vi "IdentifyChange.vi"(8 "error in (no error)":errorcluster, 9 "NewVal":T2 {"Hardware"."Logical Instrument"."Watchdog"."Interval (s)" min=1.0 max=360.0; "Hardware"."Logical Instrument"."Safety Trips"."Pmax Sink Time (s)" min=-1.0; "Hardware"."Logical Instrument"."Safety Trips"."Pmax Sink (W)" min=0.0 format="%#_7g"; "Hardware"."Logical Instrument"."Safety Trips"."Pmax Source Time (s)" min=-1.0; "Hardware"."Logical Instrument"."Safety Trips"."Pmax Source (W)" min=0.0 format="%#_7g"; "Hardware"."Logical Instrument"."Safety Trips"."Absolute Curr Peak" min=0.0; "Hardware"."Logical Instrument"."Safety Trips"."Imax Sink Time (s)" min=-1.0; "Hardware"."Logical Instrument"."Safety Trips"."Imax Sink (A)" min=0.0; "Hardware"."Logical Instrument"."Safety Trips"."Imax Source Time (s)" min=-1.0; "Hardware"."Logical Instrument"."Safety Trips"."Imax Source (A)" min=0.0; "Hardware"."Logical Instrument"."Safety Trips"."Absolute Volt Peak" min=0.0; "Hardware"."Logical Instrument"."Safety Trips"."Vmax Time (s)" min=-1.0; "Hardware"."Logical Instrument"."Safety Trips"."Vmax (V)" min=0.0; "Hardware"."Logical Instrument"."Safety Trips"."Vmin Time (s)" min=-1.0; "Hardware"."Logical Instrument"."Safety Trips"."Vmin (V)" min=0.0; "Hardware"."Logical Instrument"."Aperture (cycles)" min=1 max=64; "Hardware"."Logical Instrument"."FreqOut (Hz)" min=0.0 max=100.0; "Hardware"."Logical Instrument"."Slew Rates"."Phase Angle Min (Deg/s)" min=0.0; "Hardware"."Logical Instrument"."Slew Rates"."Phase Angle Max (Deg/s)" min=0.0; "Hardware"."Logical Instrument"."Slew Rates"."Freq Min (Hz/s)" min=0.0; "Hardware"."Logical Instrument"."Slew Rates"."Freq Max (Hz/s)" min=0.0; "Hardware"."Logical Instrument"."Slew Rates"."Pmax (W/s)" min=0.0; "Hardware"."Logical Instrument"."Slew Rates"."Pmin (W/s)" min=0.0; "Hardware"."Logical Instrument"."Slew Rates"."Imax (A/s)" min=0.0; "Hardware"."Logical Instrument"."Slew Rates"."Vmax (V/s)" min=0.0; "Hardware"."Logical Instrument"."Slew Rates"."Imin (A/s)" min=0.0; "Hardware"."Logical Instrument"."Slew Rates"."Vmin (V/s)" min=0.0; "Hardware"."Logical Instrument"."Phases"."Change at (Deg)" min=0.0; "Hardware"."Logical Instrument"."Phases"."C-Angle (Deg)" min=0.0; "Hardware"."Logical Instrument"."Phases"."B-Angle (Deg)" min=0.0; "Hardware"."Logical Instrument"."Phases"."C-Volts (V)" min=0.0; "Hardware"."Logical Instrument"."Phases"."B-Volts (V)" min=0.0; "Hardware"."Logical Instrument"."Phases"."A-Volts (V)" min=0.0; "Hardware"."Logical Instrument"."Vout (V)" min=0.0; "Hardware"."Mode" items=["3-Phase AC"=0, "AC"=1, "DC"=2, "AC - AC"=7, "AC - DC"=8, "DC - AC"=11, "DC - DC"=12, "2-Phase AC - AC"=5, "2-Phase AC - DC"=6, "AC - AC - AC"=3, "DC - DC - DC"=4, "AC - AC - DC"=9, "AC - DC - DC"=10, "AC - DC - AC"=13, "DC - AC - AC"=14, "DC - AC - DC"=15]}, 10 "OldVal":T2 {"Hardware"."Logical Instrument"."Watchdog"."Interval (s)" min=1.0 max=360.0; "Hardware"."Logical Instrument"."Safety Trips"."Pmax Sink Time (s)" min=-1.0; "Hardware"."Logical Instrument"."Safety Trips"."Pmax Sink (W)" min=0.0 format="%#_7g"; "Hardware"."Logical Instrument"."Safety Trips"."Pmax Source Time (s)" min=-1.0; "Hardware"."Logical Instrument"."Safety Trips"."Pmax Source (W)" min=0.0 format="%#_7g"; "Hardware"."Logical Instrument"."Safety Trips"."Absolute Curr Peak" min=0.0; "Hardware"."Logical Instrument"."Safety Trips"."Imax Sink Time (s)" min=-1.0; "Hardware"."Logical Instrument"."Safety Trips"."Imax Sink (A)" min=0.0; "Hardware"."Logical Instrument"."Safety Trips"."Imax Source Time (s)" min=-1.0; "Hardware"."Logical Instrument"."Safety Trips"."Imax Source (A)" min=0.0; "Hardware"."Logical Instrument"."Safety Trips"."Absolute Volt Peak" min=0.0; "Hardware"."Logical Instrument"."Safety Trips"."Vmax Time (s)" min=-1.0; "Hardware"."Logical Instrument"."Safety Trips"."Vmax (V)" min=0.0; "Hardware"."Logical Instrument"."Safety Trips"."Vmin Time (s)" min=-1.0; "Hardware"."Logical Instrument"."Safety Trips"."Vmin (V)" min=0.0; "Hardware"."Logical Instrument"."Aperture (cycles)" min=1 max=64; "Hardware"."Logical Instrument"."FreqOut (Hz)" min=0.0 max=100.0; "Hardware"."Logical Instrument"."Slew Rates"."Phase Angle Min (Deg/s)" min=0.0; "Hardware"."Logical Instrument"."Slew Rates"."Phase Angle Max (Deg/s)" min=0.0; "Hardware"."Logical Instrument"."Slew Rates"."Freq Min (Hz/s)" min=0.0; "Hardware"."Logical Instrument"."Slew Rates"."Freq Max (Hz/s)" min=0.0; "Hardware"."Logical Instrument"."Slew Rates"."Pmax (W/s)" min=0.0; "Hardware"."Logical Instrument"."Slew Rates"."Pmin (W/s)" min=0.0; "Hardware"."Logical Instrument"."Slew Rates"."Imax (A/s)" min=0.0; "Hardware"."Logical Instrument"."Slew Rates"."Vmax (V/s)" min=0.0; "Hardware"."Logical Instrument"."Slew Rates"."Imin (A/s)" min=0.0; "Hardware"."Logical Instrument"."Slew Rates"."Vmin (V/s)" min=0.0; "Hardware"."Logical Instrument"."Phases"."Change at (Deg)" min=0.0; "Hardware"."Logical Instrument"."Phases"."C-Angle (Deg)" min=0.0; "Hardware"."Logical Instrument"."Phases"."B-Angle (Deg)" min=0.0; "Hardware"."Logical Instrument"."Phases"."C-Volts (V)" min=0.0; "Hardware"."Logical Instrument"."Phases"."B-Volts (V)" min=0.0; "Hardware"."Logical Instrument"."Phases"."A-Volts (V)" min=0.0; "Hardware"."Logical Instrument"."Vout (V)" min=0.0; "Hardware"."Mode" items=["3-Phase AC"=0, "AC"=1, "DC"=2, "AC - AC"=7, "AC - DC"=8, "DC - AC"=11, "DC - DC"=12, "2-Phase AC - AC"=5, "2-Phase AC - DC"=6, "AC - AC - AC"=3, "DC - DC - DC"=4, "AC - AC - DC"=9, "AC - DC - DC"=10, "AC - DC - AC"=13, "DC - AC - AC"=14, "DC - AC - DC"=15]}, 11 "Settings In":T2 {"Hardware"."Logical Instrument"."Watchdog"."Interval (s)" min=1.0 max=360.0; "Hardware"."Logical Instrument"."Safety Trips"."Pmax Sink Time (s)" min=-1.0; "Hardware"."Logical Instrument"."Safety Trips"."Pmax Sink (W)" min=0.0 format="%#_7g"; "Hardware"."Logical Instrument"."Safety Trips"."Pmax Source Time (s)" min=-1.0; "Hardware"."Logical Instrument"."Safety Trips"."Pmax Source (W)" min=0.0 format="%#_7g"; "Hardware"."Logical Instrument"."Safety Trips"."Absolute Curr Peak" min=0.0; "Hardware"."Logical Instrument"."Safety Trips"."Imax Sink Time (s)" min=-1.0; "Hardware"."Logical Instrument"."Safety Trips"."Imax Sink (A)" min=0.0; "Hardware"."Logical Instrument"."Safety Trips"."Imax Source Time (s)" min=-1.0; "Hardware"."Logical Instrument"."Safety Trips"."Imax Source (A)" min=0.0; "Hardware"."Logical Instrument"."Safety Trips"."Absolute Volt Peak" min=0.0; "Hardware"."Logical Instrument"."Safety Trips"."Vmax Time (s)" min=-1.0; "Hardware"."Logical Instrument"."Safety Trips"."Vmax (V)" min=0.0; "Hardware"."Logical Instrument"."Safety Trips"."Vmin Time (s)" min=-1.0; "Hardware"."Logical Instrument"."Safety Trips"."Vmin (V)" min=0.0; "Hardware"."Logical Instrument"."Aperture (cycles)" min=1 max=64; "Hardware"."Logical Instrument"."FreqOut (Hz)" min=0.0 max=100.0; "Hardware"."Logical Instrument"."Slew Rates"."Phase Angle Min (Deg/s)" min=0.0; "Hardware"."Logical Instrument"."Slew Rates"."Phase Angle Max (Deg/s)" min=0.0; "Hardware"."Logical Instrument"."Slew Rates"."Freq Min (Hz/s)" min=0.0; "Hardware"."Logical Instrument"."Slew Rates"."Freq Max (Hz/s)" min=0.0; "Hardware"."Logical Instrument"."Slew Rates"."Pmax (W/s)" min=0.0; "Hardware"."Logical Instrument"."Slew Rates"."Pmin (W/s)" min=0.0; "Hardware"."Logical Instrument"."Slew Rates"."Imax (A/s)" min=0.0; "Hardware"."Logical Instrument"."Slew Rates"."Vmax (V/s)" min=0.0; "Hardware"."Logical Instrument"."Slew Rates"."Imin (A/s)" min=0.0; "Hardware"."Logical Instrument"."Slew Rates"."Vmin (V/s)" min=0.0; "Hardware"."Logical Instrument"."Phases"."Change at (Deg)" min=0.0; "Hardware"."Logical Instrument"."Phases"."C-Angle (Deg)" min=0.0; "Hardware"."Logical Instrument"."Phases"."B-Angle (Deg)" min=0.0; "Hardware"."Logical Instrument"."Phases"."C-Volts (V)" min=0.0; "Hardware"."Logical Instrument"."Phases"."B-Volts (V)" min=0.0; "Hardware"."Logical Instrument"."Phases"."A-Volts (V)" min=0.0; "Hardware"."Logical Instrument"."Vout (V)" min=0.0; "Hardware"."Mode" items=["3-Phase AC"=0, "AC"=1, "DC"=2, "AC - AC"=7, "AC - DC"=8, "DC - AC"=11, "DC - DC"=12, "2-Phase AC - AC"=5, "2-Phase AC - DC"=6, "AC - AC - AC"=3, "DC - DC - DC"=4, "AC - AC - DC"=9, "AC - DC - DC"=10, "AC - DC - AC"=13, "DC - AC - AC"=14, "DC - AC - DC"=15]}) -> (0 "error out":errorcluster, 1 "Instrument Index":i32, 2 "Ctrl Label":string, 3 "Settings Out":T2 {"Hardware"."Logical Instrument"."Watchdog"."Interval (s)" min=1.0 max=360.0; "Hardware"."Logical Instrument"."Safety Trips"."Pmax Sink Time (s)" min=-1.0; "Hardware"."Logical Instrument"."Safety Trips"."Pmax Sink (W)" min=0.0 format="%#_7g"; "Hardware"."Logical Instrument"."Safety Trips"."Pmax Source Time (s)" min=-1.0; "Hardware"."Logical Instrument"."Safety Trips"."Pmax Source (W)" min=0.0 format="%#_7g"; "Hardware"."Logical Instrument"."Safety Trips"."Absolute Curr Peak" min=0.0; "Hardware"."Logical Instrument"."Safety Trips"."Imax Sink Time (s)" min=-1.0; "Hardware"."Logical Instrument"."Safety Trips"."Imax Sink (A)" min=0.0; "Hardware"."Logical Instrument"."Safety Trips"."Imax Source Time (s)" min=-1.0; "Hardware"."Logical Instrument"."Safety Trips"."Imax Source (A)" min=0.0; "Hardware"."Logical Instrument"."Safety Trips"."Absolute Volt Peak" min=0.0; "Hardware"."Logical Instrument"."Safety Trips"."Vmax Time (s)" min=-1.0; "Hardware"."Logical Instrument"."Safety Trips"."Vmax (V)" min=0.0; "Hardware"."Logical Instrument"."Safety Trips"."Vmin Time (s)" min=-1.0; "Hardware"."Logical Instrument"."Safety Trips"."Vmin (V)" min=0.0; "Hardware"."Logical Instrument"."Aperture (cycles)" min=1 max=64; "Hardware"."Logical Instrument"."FreqOut (Hz)" min=0.0 max=100.0; "Hardware"."Logical Instrument"."Slew Rates"."Phase Angle Min (Deg/s)" min=0.0; "Hardware"."Logical Instrument"."Slew Rates"."Phase Angle Max (Deg/s)" min=0.0; "Hardware"."Logical Instrument"."Slew Rates"."Freq Min (Hz/s)" min=0.0; "Hardware"."Logical Instrument"."Slew Rates"."Freq Max (Hz/s)" min=0.0; "Hardware"."Logical Instrument"."Slew Rates"."Pmax (W/s)" min=0.0; "Hardware"."Logical Instrument"."Slew Rates"."Pmin (W/s)" min=0.0; "Hardware"."Logical Instrument"."Slew Rates"."Imax (A/s)" min=0.0; "Hardware"."Logical Instrument"."Slew Rates"."Vmax (V/s)" min=0.0; "Hardware"."Logical Instrument"."Slew Rates"."Imin (A/s)" min=0.0; "Hardware"."Logical Instrument"."Slew Rates"."Vmin (V/s)" min=0.0; "Hardware"."Logical Instrument"."Phases"."Change at (Deg)" min=0.0; "Hardware"."Logical Instrument"."Phases"."C-Angle (Deg)" min=0.0; "Hardware"."Logical Instrument"."Phases"."B-Angle (Deg)" min=0.0; "Hardware"."Logical Instrument"."Phases"."C-Volts (V)" min=0.0; "Hardware"."Logical Instrument"."Phases"."B-Volts (V)" min=0.0; "Hardware"."Logical Instrument"."Phases"."A-Volts (V)" min=0.0; "Hardware"."Logical Instrument"."Vout (V)" min=0.0; "Hardware"."Mode" items=["3-Phase AC"=0, "AC"=1, "DC"=2, "AC - AC"=7, "AC - DC"=8, "DC - AC"=11, "DC - DC"=12, "2-Phase AC - AC"=5, "2-Phase AC - DC"=6, "AC - AC - AC"=3, "DC - DC - DC"=4, "AC - AC - DC"=9, "AC - DC - DC"=10, "AC - DC - AC"=13, "DC - AC - AC"=14, "DC - AC - DC"=15]})   [LabVIEW 2018, in "AcPwrPlugins.lvlib" / "NHRGridSim.lvclass"]
doc: "When the user makes any changes in the NHRGrid \"Settings\", this VI identifies which specific control was changed, and from which logical instrument."
uses:
  NHRGridSim.lvclass
  TypeDefs/NHRGrid_Device(s)Settings.ctl
  TypeDefs/NHRGrid_Hardware.ctl
  TypeDefs/NHRGrid_Modes.ctl
  TypeDefs/NHRGrid_Logical_Instrument.ctl
  TypeDefs/NHRGrid_InstrumentCluster.ctl
  TypeDefs/NHRGrid_Phases.ctl
  TypeDefs/NHRGrid_SlewRates.ctl
  TypeDefs/NHRGrid_Ranges.ctl
  TypeDefs/NHRGrid_SafetyTrips.ctl
  TypeDefs/NHRGrid_Watchdog.ctl
  TypeDefs/NHRGrid_ItemCheck.ctl
panel:
  in  "Tab Control":T1(tab)
  # "Voltages (L-N)"
  # "Voltages (L-N)"
  # "Voltages (L-N)"
  # "Voltages (L-N)"
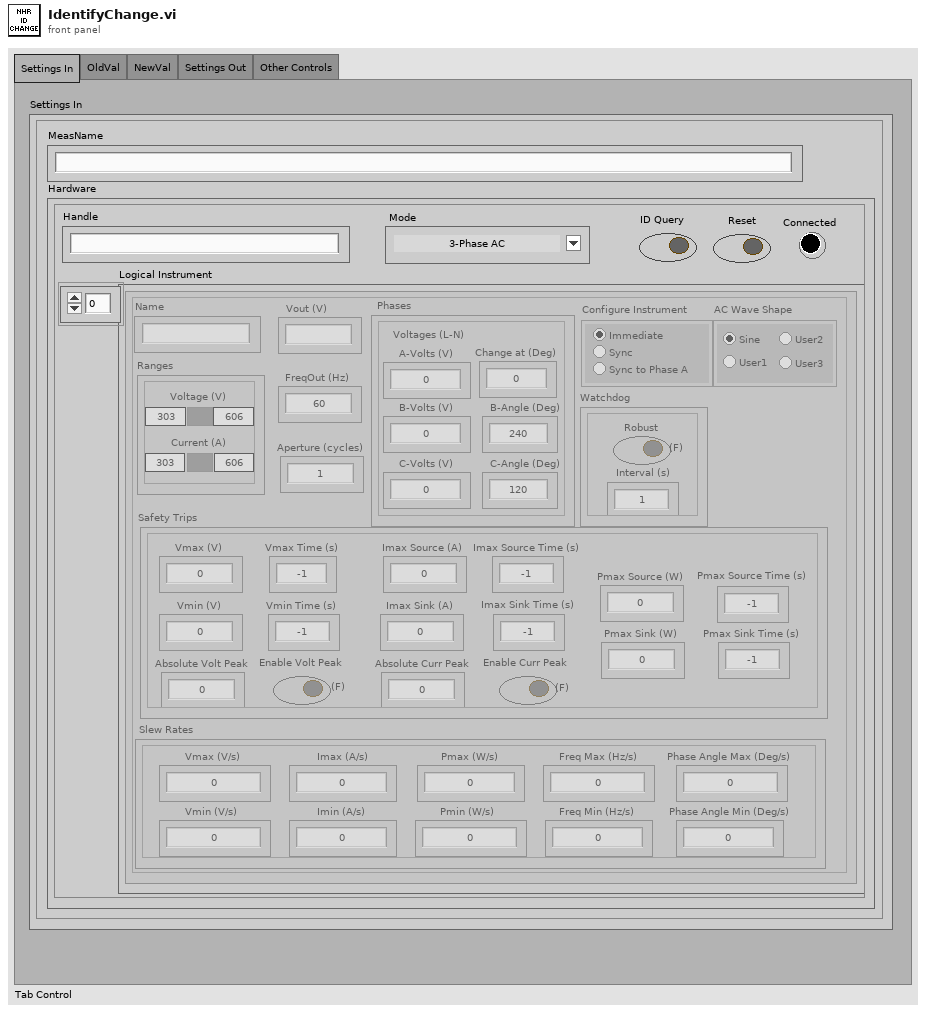
[diagram p1: front panel]
types:
  T1 = enum32{"Settings In", "OldVal", "NewVal", "Settings Out", "Other Controls"}
  T2 = typedef "AcPwrPlugins.lvlib/NHRGridSim.lvclass/NHRGrid_Device(s)Settings.ctl" = cluster{"MeasName":string, "Hardware":T3}
  T3 = typedef "AcPwrPlugins.lvlib/NHRGridSim.lvclass/NHRGrid_Hardware.ctl" = cluster{"Handle":string, "Reset":bool, "Mode":T4, "ID Query":bool, "Connected":bool, "Logical Instrument":T5}
  T4 = typedef "AcPwrPlugins.lvlib/NHRGridSim.lvclass/NHRGrid_Modes.ctl" = u8
  T5 = typedef "AcPwrPlugins.lvlib/NHRGridSim.lvclass/NHRGrid_Logical_Instrument.ctl" = T6[]
  T6 = typedef "AcPwrPlugins.lvlib/NHRGridSim.lvclass/NHRGrid_InstrumentCluster.ctl" = cluster{"Name":string, "Vout (V)":dbl, "VType":string, "Phases":T7, "Slew Rates":T8, "FreqOut (Hz)":dbl, "Aperture (cycles)":i32, "Configure Instrument":enum32{"Conf1", "Conf2", "Conf3"}, "AC Wave Shape":enum32{"Sine", "User1", "User2", "User3"}, "Ranges":T9, "Safety Trips":T10, "Watchdog":T11}
  T7 = typedef "AcPwrPlugins.lvlib/NHRGridSim.lvclass/NHRGrid_Phases.ctl" = cluster{"A-Volts (V)":dbl, "B-Volts (V)":dbl, "C-Volts (V)":dbl, "Change at (Deg)":dbl, "B-Angle (Deg)":dbl, "C-Angle (Deg)":dbl}
  T8 = typedef "AcPwrPlugins.lvlib/NHRGridSim.lvclass/NHRGrid_SlewRates.ctl" = cluster{"Vmax (V/s)":dbl, "Vmin (V/s)":dbl, "Imax (A/s)":dbl, "Imin (A/s)":dbl, "Pmax (W/s)":dbl, "Pmin (W/s)":dbl, "Freq Max (Hz/s)":dbl, "Freq Min (Hz/s)":dbl, "Phase Angle Max (Deg/s)":dbl, "Phase Angle Min (Deg/s)":dbl}
  T9 = typedef "AcPwrPlugins.lvlib/NHRGridSim.lvclass/NHRGrid_Ranges.ctl" = cluster{"Voltage (V)":bool, "VHi":dbl, "Current (A)":bool, "CLo":dbl, "CHi":dbl, "VLo":dbl}
  T10 = typedef "AcPwrPlugins.lvlib/NHRGridSim.lvclass/NHRGrid_SafetyTrips.ctl" = cluster{"Vmax (V)":dbl, "Vmin (V)":dbl, "Vmax Time (s)":dbl, "Vmin Time (s)":dbl, "Imax Source (A)":dbl, "Imax Sink (A)":dbl, "Imax Source Time (s)":dbl, "Imax Sink Time (s)":dbl, "Pmax Source (W)":dbl, "Pmax Sink (W)":dbl, "Pmax Source Time (s)":dbl, "Pmax Sink Time (s)":dbl, "Absolute Volt Peak":dbl, "Enable Volt Peak":bool, "Absolute Curr Peak":dbl, "Enable Curr Peak":bool, "Setting t":string, "Recomm t 2":string}
  T11 = typedef "AcPwrPlugins.lvlib/NHRGridSim.lvclass/NHRGrid_Watchdog.ctl" = cluster{"Robust":bool, "Interval (s)":dbl}
  T12 = typedef "AcPwrPlugins.lvlib/NHRGridSim.lvclass/NHRGrid_ItemCheck.ctl" = enum16{"Handle", "Mode", "ID Query", "Reset", "Name", "Vout", "RangeV Lo", "RangeV Hi", "RangeV Sw", "RangeC Lo", "RangeC Hi", "RangeC Sw", "FreqOut", "Aperture", "PhaseA V", "PhaseB V", "PhaseC V", "PhaseB Ang", "PhaseC Ang", "Change at", "Configure", "AC Wave", "Watch Robust", "Watch Int", "Safe Vmax", "Safe Vmin", "Safe VmaxT", "Safe VminT", "Safe I Sour", "Safe I Sink", "Safe I SourT", "Safe I SinkT", "Safe P Sour", "Safe P Sink", "Safe P SourT", "Safe P SinkT", "Abs V Peak", "Enab V Peak", "Abs I Peak", "Enab I Peak", "Slew Vmax", "Slew v min", "Slew Imax", "Slew Imin", "Slew Pmax", "Slew Pmin", "Slew Fmax", "Slew Fmin", "Slew AngMax", "Slew AngMin", "Exit", "Update", "Enable"}
  T13 = cluster{"MeasName":bool, "Hardware":cluster{"Handle":bool, "Reset":bool, "Mode":bool, "ID Query":bool, "Connected":bool, "Logical Instrument":cluster{"Name":bool, "Vout (V)":bool, "VType":bool, "Phases":cluster{"A-Volts (V)":bool, "B-Volts (V)":bool, "C-Volts (V)":bool, "Change at (Deg)":bool, "B-Angle (Deg)":bool, "C-Angle (Deg)":bool}, "Slew Rates":cluster{"Vmax (V/s)":bool, "Vmin (V/s)":bool, "Imax (A/s)":bool, "Imin (A/s)":bool, "Pmax (W/s)":bool, "Pmin (W/s)":bool, "Freq Max (Hz/s)":bool, "Freq Min (Hz/s)":bool, "Phase Angle Max (Deg/s)":bool, "Phase Angle Min (Deg/s)":bool}, "FreqOut (Hz)":bool, "Aperture (cycles)":bool, "Configure Instrument":bool, "AC Wave Shape":bool, "Ranges":cluster{"Voltage (V)":bool, "VHi":bool, "Current (A)":bool, "CLo":bool, "CHi":bool, "VLo":bool}, "Safety Trips":cluster{"Vmax (V)":bool, "Vmin (V)":bool, "Vmax Time (s)":bool, "Vmin Time (s)":bool, "Imax Source (A)":bool, "Imax Sink (A)":bool, "Imax Source Time (s)":bool, "Imax Sink Time (s)":bool, "Pmax Source (W)":bool, "Pmax Sink (W)":bool, "Pmax Source Time (s)":bool, "Pmax Sink Time (s)":bool, "Absolute Volt Peak":bool, "Enable Volt Peak":bool, "Absolute Curr Peak":bool, "Enable Curr Peak":bool, "Setting t":bool, "Recomm t 2":bool}, "Watchdog":cluster{"Robust":bool, "Interval (s)":bool}}[]}}
  T14 = cluster{"Handle":bool, "Reset":bool, "Mode":bool, "ID Query":bool, "Connected":bool, "Logical Instrument":cluster{"Name":bool, "Vout (V)":bool, "VType":bool, "Phases":cluster{"A-Volts (V)":bool, "B-Volts (V)":bool, "C-Volts (V)":bool, "Change at (Deg)":bool, "B-Angle (Deg)":bool, "C-Angle (Deg)":bool}, "Slew Rates":cluster{"Vmax (V/s)":bool, "Vmin (V/s)":bool, "Imax (A/s)":bool, "Imin (A/s)":bool, "Pmax (W/s)":bool, "Pmin (W/s)":bool, "Freq Max (Hz/s)":bool, "Freq Min (Hz/s)":bool, "Phase Angle Max (Deg/s)":bool, "Phase Angle Min (Deg/s)":bool}, "FreqOut (Hz)":bool, "Aperture (cycles)":bool, "Configure Instrument":bool, "AC Wave Shape":bool, "Ranges":cluster{"Voltage (V)":bool, "VHi":bool, "Current (A)":bool, "CLo":bool, "CHi":bool, "VLo":bool}, "Safety Trips":cluster{"Vmax (V)":bool, "Vmin (V)":bool, "Vmax Time (s)":bool, "Vmin Time (s)":bool, "Imax Source (A)":bool, "Imax Sink (A)":bool, "Imax Source Time (s)":bool, "Imax Sink Time (s)":bool, "Pmax Source (W)":bool, "Pmax Sink (W)":bool, "Pmax Source Time (s)":bool, "Pmax Sink Time (s)":bool, "Absolute Volt Peak":bool, "Enable Volt Peak":bool, "Absolute Curr Peak":bool, "Enable Curr Peak":bool, "Setting t":bool, "Recomm t 2":bool}, "Watchdog":cluster{"Robust":bool, "Interval (s)":bool}}[]}
  T15 = cluster{"Name":bool, "Vout (V)":bool, "VType":bool, "Phases":cluster{"A-Volts (V)":bool, "B-Volts (V)":bool, "C-Volts (V)":bool, "Change at (Deg)":bool, "B-Angle (Deg)":bool, "C-Angle (Deg)":bool}, "Slew Rates":cluster{"Vmax (V/s)":bool, "Vmin (V/s)":bool, "Imax (A/s)":bool, "Imin (A/s)":bool, "Pmax (W/s)":bool, "Pmin (W/s)":bool, "Freq Max (Hz/s)":bool, "Freq Min (Hz/s)":bool, "Phase Angle Max (Deg/s)":bool, "Phase Angle Min (Deg/s)":bool}, "FreqOut (Hz)":bool, "Aperture (cycles)":bool, "Configure Instrument":bool, "AC Wave Shape":bool, "Ranges":cluster{"Voltage (V)":bool, "VHi":bool, "Current (A)":bool, "CLo":bool, "CHi":bool, "VLo":bool}, "Safety Trips":cluster{"Vmax (V)":bool, "Vmin (V)":bool, "Vmax Time (s)":bool, "Vmin Time (s)":bool, "Imax Source (A)":bool, "Imax Sink (A)":bool, "Imax Source Time (s)":bool, "Imax Sink Time (s)":bool, "Pmax Source (W)":bool, "Pmax Sink (W)":bool, "Pmax Source Time (s)":bool, "Pmax Sink Time (s)":bool, "Absolute Volt Peak":bool, "Enable Volt Peak":bool, "Absolute Curr Peak":bool, "Enable Curr Peak":bool, "Setting t":bool, "Recomm t 2":bool}, "Watchdog":cluster{"Robust":bool, "Interval (s)":bool}}[]
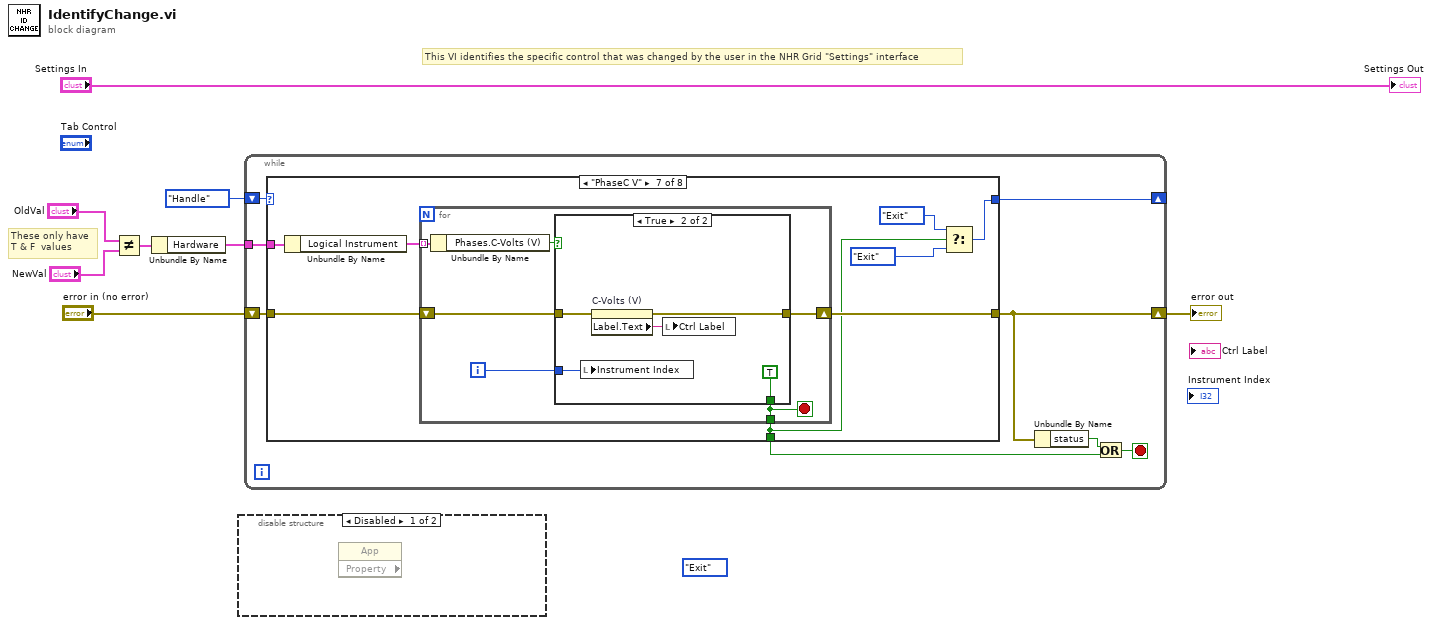
[diagram p0: block diagram]
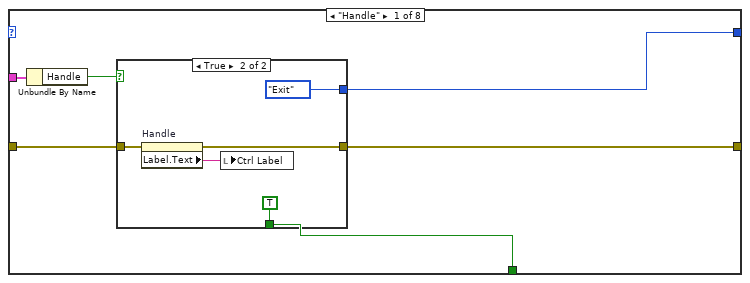
[diagram p3: hidden frame]
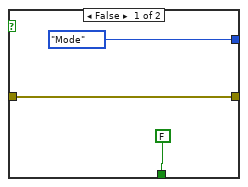
[diagram p4: hidden frame]
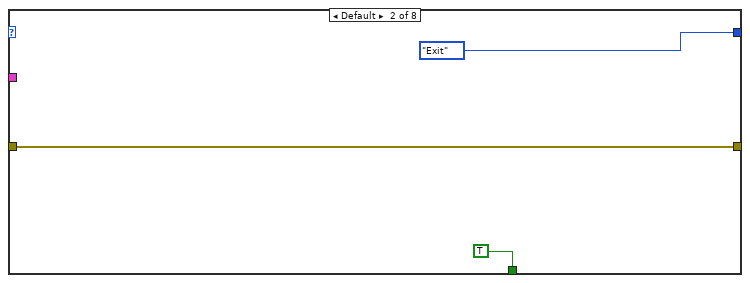
[diagram p5: hidden frame]
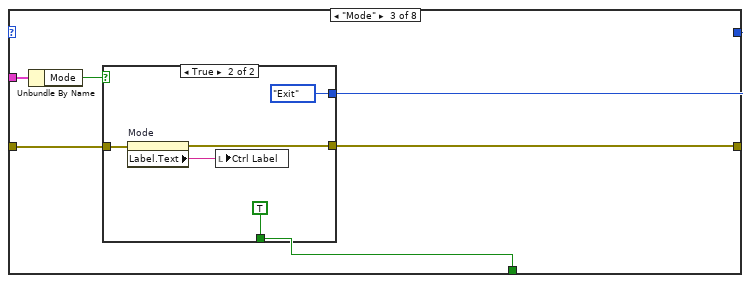
[diagram p6: hidden frame]
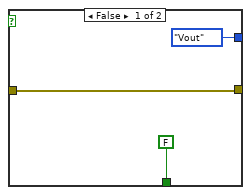
[diagram p7: hidden frame]
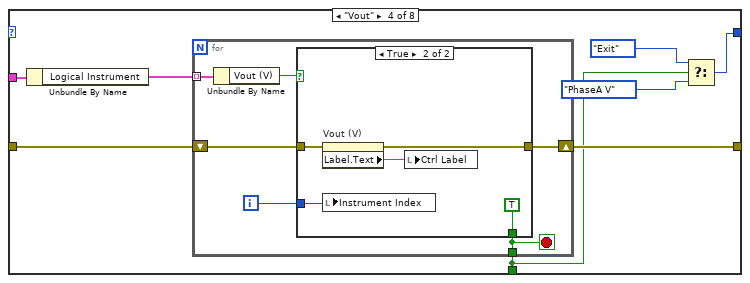
[diagram p8: hidden frame]
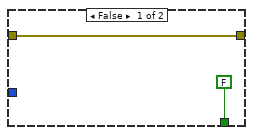
[diagram p9: hidden frame]
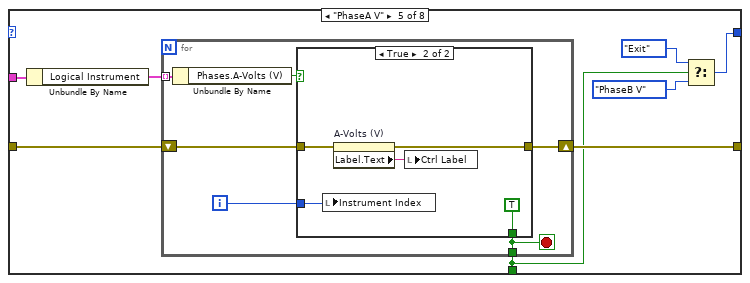
[diagram p10: hidden frame]
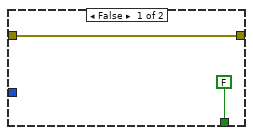
[diagram p11: hidden frame]
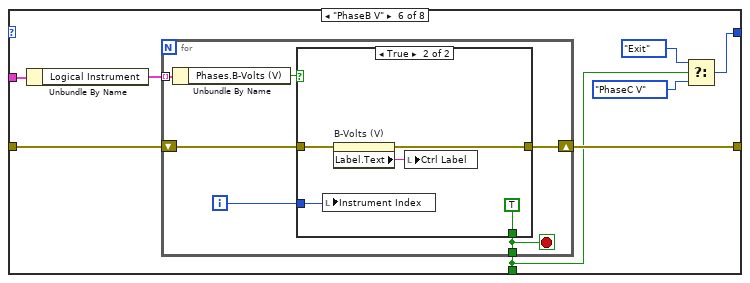
[diagram p12: hidden frame]
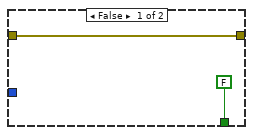
[diagram p13: hidden frame]
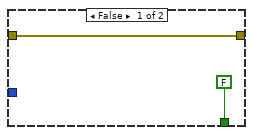
[diagram p14: hidden frame]
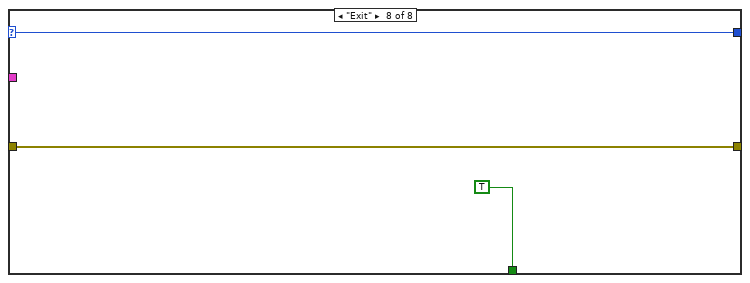
[diagram p15: hidden frame]
diagram:
  (unwired) NHRGrid_ItemCheck."Exit" ("AcPwrPlugins.lvlib:NhRegenGridSim.lvclass:ConfigDevicesTypeDef")
  # "These only have T & F  values"
  # "This VI identifies the specific control that was changed by the user in the NHR Grid \"Settings\" interface"
  n1 = Not Equal?(x="OldVal", y="NewVal") -> (x != y?=w3:T13)
  n2 = Unbundle By Name(w3) -> ("Hardware"=w6:T14)
  n3 = disable-structure shown="Disabled" {
    frame Disabled {
      n4 = property class="App" props=[]() -> ()  [unwired: 2 in, 3 out]
    }
    frame Enabled {
    }
  }
  n5 = while {
    tunnel: w6 -> [w12]
    shift-right: [w10] -> _
    shift-left: NHRGrid_ItemCheck."Handle" ("AcPwrPlugins.lvlib:NhRegenGridSim.lvclass:ConfigDevicesTypeDef") -> [w11]
    shift-right: [w15] -> w4
    shift-left: "error in (no error)" -> [w16]
    stop <- w14 stop-if-true
    n6 = case shown="\"PhaseC V\"" w11 {
      selector: w11 -> [_ _ _ _ _ _ _ w134]
      tunnel: [w17 TRUE w34 w51 w72 w93 w114 TRUE] -> w13
      tunnel: [w20 NHRGrid_ItemCheck."Exit" ("AcPwrPlugins.lvlib:NhRegenGridSim.lvclass:ConfigDevicesTypeDef") w37 w49 w70 w91 w112 w134] -> w10
      tunnel: w12 -> [w22 _ w38 w53 w74 w95 w116 _]
      tunnel: w16 -> [w19 w32 w36 w55 w76 w97 w118 w132]
      tunnel: [w18 w32 w35 w54 w75 w96 w117 w132] -> w15
      frame "Handle" {
        n7 = Unbundle By Name(w22) -> ("Handle"=w21:bool)
        n8 = case shown="True" w21 {
          tunnel: [NHRGrid_ItemCheck."Mode" ("AcPwrPlugins.lvlib:NhRegenGridSim.lvclass:ConfigDevicesTypeDef") NHRGrid_ItemCheck."Exit" ("AcPwrPlugins.lvlib:NHRGridSim.lvclass:NHRGrid_ItemCheck")] -> w20
          tunnel: [FALSE TRUE] -> w17
          tunnel: w19 -> [w24 w28]
          tunnel: [w24 w27] -> w18
          frame False {
          }
          frame True {
            n9 = property on="Handle" class="Str"(error in=w28) -> (error out=w27:errorcluster, "Label.Text"=w29:string)  [unwired: 1 in, 1 out]
            n10 = local write "Ctrl Label"(w29) -> ()
          }
        }
      }
      frame Default {
      }
      frame "Mode" {
        n11 = Unbundle By Name(w38) -> ("Mode"=w39:bool)
        n12 = case shown="True" w39 {
          tunnel: [NHRGrid_ItemCheck."Vout" ("AcPwrPlugins.lvlib:NhRegenGridSim.lvclass:ConfigDevicesTypeDef") NHRGrid_ItemCheck."Exit" ("AcPwrPlugins.lvlib:NhRegenGridSim.lvclass:ConfigDevicesTypeDef")] -> w37
          tunnel: [FALSE TRUE] -> w34
          tunnel: w36 -> [w41 w45]
          tunnel: [w41 w44] -> w35
          frame False {
          }
          frame True {
            n13 = property on="Mode" class="Ring (strict)"(error in=w45) -> (error out=w44:errorcluster, "Label.Text"=w46:string)  [unwired: 1 in, 1 out]
            n14 = local write "Ctrl Label"(w46) -> ()
          }
        }
      }
      frame "Vout" {
        n15 = Unbundle By Name(w53) -> ("Logical Instrument"=w52:T15)
        n16 = for {
          shift-right: [w60] -> w54
          shift-left: w55 -> [w61]
          tunnel: w52 -> [w59] mode=indexing
          tunnel: [w56] -> w51
          i -> [w57]
          stop <- w56 stop-if-true
          n17 = Unbundle By Name(w59) -> ("Vout (V)"=w58:bool)
          n18 = case shown="True" w58 {
            tunnel: [FALSE TRUE] -> w56
            tunnel: w61 -> [w62 w65]
            tunnel: [w62 w66] -> w60
            tunnel: w57 -> [_ w67]
            frame False {
            }
            frame True {
              n19 = property on="Vout (V)" class="DigNum (strict)"(error in=w65) -> (error out=w66:errorcluster, "Label.Text"=w64:string)  [unwired: 1 in, 1 out]
              n20 = local write "Instrument Index"(w67) -> ()
              n21 = local write "Ctrl Label"(w64) -> ()
            }
          }
        }
        n22 = Select(t=NHRGrid_ItemCheck."Exit" ("AcPwrPlugins.lvlib:NhRegenGridSim.lvclass:ConfigDevicesTypeDef"), s=w51, f=NHRGrid_ItemCheck."PhaseA V" ("AcPwrPlugins.lvlib:NhRegenGridSim.lvclass:ConfigDevicesTypeDef")) -> (s? t:f=w49:T12)
      }
      frame "PhaseA V" {
        n23 = Unbundle By Name(w74) -> ("Logical Instrument"=w73:T15)
        n24 = for {
          shift-right: [w81] -> w75
          shift-left: w76 -> [w82]
          tunnel: w73 -> [w80] mode=indexing
          tunnel: [w77] -> w72
          i -> [w78]
          stop <- w77 stop-if-true
          n25 = Unbundle By Name(w80) -> ("Phases.A-Volts (V)"=w79:bool)
          n26 = case shown="True" w79 {
            tunnel: [FALSE TRUE] -> w77
            tunnel: w82 -> [w83 w86]
            tunnel: [w83 w87] -> w81
            tunnel: w78 -> [_ w88]
            frame False {
            }
            frame True {
              n27 = local write "Instrument Index"(w88) -> ()
              n28 = property on="A-Volts (V)" class="DigNum (strict)"(error in=w86) -> (error out=w87:errorcluster, "Label.Text"=w85:string)  [unwired: 1 in, 1 out]
              n29 = local write "Ctrl Label"(w85) -> ()
            }
          }
        }
        n30 = Select(t=NHRGrid_ItemCheck."Exit" ("AcPwrPlugins.lvlib:NhRegenGridSim.lvclass:ConfigDevicesTypeDef"), s=w72, f=NHRGrid_ItemCheck."PhaseB V" ("AcPwrPlugins.lvlib:NhRegenGridSim.lvclass:ConfigDevicesTypeDef")) -> (s? t:f=w70:T12)
      }
      frame "PhaseB V" {
        n31 = Unbundle By Name(w95) -> ("Logical Instrument"=w94:T15)
        n32 = for {
          shift-right: [w102] -> w96
          shift-left: w97 -> [w103]
          tunnel: w94 -> [w101] mode=indexing
          tunnel: [w98] -> w93
          i -> [w99]
          stop <- w98 stop-if-true
          n33 = Unbundle By Name(w101) -> ("Phases.B-Volts (V)"=w100:bool)
          n34 = case shown="True" w100 {
            tunnel: [FALSE TRUE] -> w98
            tunnel: w103 -> [w104 w107]
            tunnel: [w104 w108] -> w102
            tunnel: w99 -> [_ w109]
            frame False {
            }
            frame True {
              n35 = local write "Instrument Index"(w109) -> ()
              n36 = property on="B-Volts (V)" class="DigNum (strict)"(error in=w107) -> (error out=w108:errorcluster, "Label.Text"=w106:string)  [unwired: 1 in, 1 out]
              n37 = local write "Ctrl Label"(w106) -> ()
            }
          }
        }
        n38 = Select(t=NHRGrid_ItemCheck."Exit" ("AcPwrPlugins.lvlib:NhRegenGridSim.lvclass:ConfigDevicesTypeDef"), s=w93, f=NHRGrid_ItemCheck."PhaseC V" ("AcPwrPlugins.lvlib:NhRegenGridSim.lvclass:ConfigDevicesTypeDef")) -> (s? t:f=w91:T12)
      }
      frame "PhaseC V" {
        n39 = Unbundle By Name(w116) -> ("Logical Instrument"=w115:T15)
        n40 = for {
          shift-right: [w123] -> w117
          shift-left: w118 -> [w124]
          tunnel: w115 -> [w122] mode=indexing
          tunnel: [w119] -> w114
          i -> [w120]
          stop <- w119 stop-if-true
          n41 = Unbundle By Name(w122) -> ("Phases.C-Volts (V)"=w121:bool)
          n42 = case shown="True" w121 {
            tunnel: [FALSE TRUE] -> w119
            tunnel: w124 -> [w125 w128]
            tunnel: [w125 w129] -> w123
            tunnel: w120 -> [_ w130]
            frame False {
            }
            frame True {
              n43 = local write "Instrument Index"(w130) -> ()
              n44 = property on="C-Volts (V)" class="DigNum (strict)"(error in=w128) -> (error out=w129:errorcluster, "Label.Text"=w127:string)  [unwired: 1 in, 1 out]
              n45 = local write "Ctrl Label"(w127) -> ()
            }
          }
        }
        n46 = Select(t=NHRGrid_ItemCheck."Exit" ("AcPwrPlugins.lvlib:NhRegenGridSim.lvclass:ConfigDevicesTypeDef"), s=w114, f=NHRGrid_ItemCheck."Exit" ("AcPwrPlugins.lvlib:NhRegenGridSim.lvclass:ConfigDevicesTypeDef")) -> (s? t:f=w112:T12)
      }
      frame "Exit" {
      }
    }
    n47 = Unbundle By Name(w15) -> ("status"=w9:bool)
    n48 = Or(x=w9, y=w13) -> (x .or. y?=w14:bool)
  }
  "error out" <- w4
  "Settings Out" <- "Settings In"
